vi "Set Error.vi"(4 "Log Error?":bool, 6 "Error Message":string, 7 "Error Codes":T1) -> (3 "Error Interface out":refnum<class "Error Interface.lvclass">)   [LabVIEW 2016, in "Stream Error.lvlib" / "Error Interface.lvclass"]
doc: "--\nCopyright © 2017 Composed SystemsI All rights reserved.\n\nAuthor: Jon McBee <jon.mcbee@composed.io>\n\nThis library is provided \"AS IS\" ,WITHOUT WARRANTIES OR\nCONDITIONS OF ANY KIND, either express or implied.\n\nComposed Systems -- composed.io\n\nStream 0.0.1.1\nJon McBee - Composed Systems\nCopyright (c) 2017, Composed Systems"
uses:
  <userlib>/Composed Systems/Stream/Error/Classes/Error Interface/Error Interface.lvclass
  <userlib>/Composed Systems/Stream/Error/Classes/Error Interface/Error Codes.ctl
  <userlib>/Composed Systems/Stream/Error/Classes/Error Interface/Error Interface.lvclass/Error Interface.ctl
  <userlib>/Composed Systems/Stream/Log/Application Log/Log Level.ctl
  <userlib>/Composed Systems/Stream/Log/Global Application Log/Global Application Log.lvclass
  <userlib>/Composed Systems/Stream/Log/Application Log/Application Log.lvclass
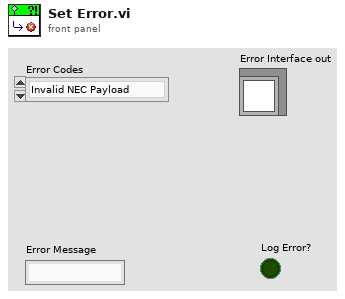
[diagram p1: front panel]
types:
  T1 = typedef "Stream Error.lvlib/Error Interface.lvclass/Error Codes.ctl" = enum16{"Invalid NEC Payload"}
  T2 = typedef "Stream Log.lvlib/Application Log.lvclass/Log Level.ctl" = enum16{"Imperative", "Major", "Minor", "Debug", "Off"}
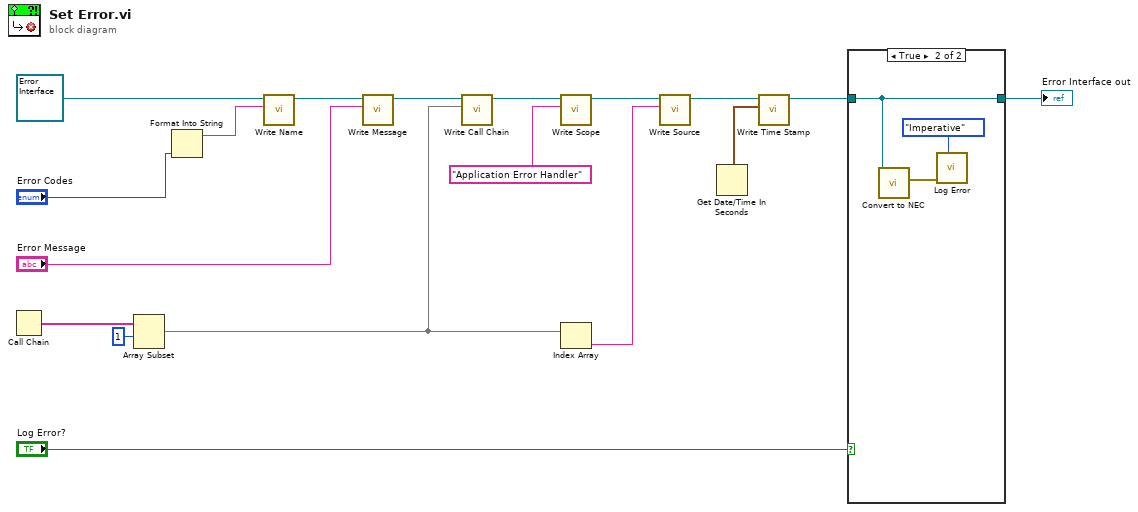
[diagram p0: block diagram]
diagram:
  n1 = Call Chain() -> (call chain=w9:string[])
  n2 = Array Subset(array=w9, index=1) -> (w5:string[])  [unwired: 1 in]
  n3 = Format Into String("Error Codes") -> (resulting string=w15:string)  [unwired: 3 in, 1 out]
  n4 = call <userlib>:"Write Name.vi"("Name"=w15, "Error Interface in"=refnum<class "Error Interface.lvclass"> refnum ("Error Interface out")) -> ("Error Interface out"=w17:refnum<class "Error Interface.lvclass">)  [unwired: 8 in, 1 out]
  n5 = call <userlib>:"Write Message.vi"("Message"="Error Message", "Error Interface in"=w17) -> ("Error Interface out"=w13:refnum<class "Error Interface.lvclass">)  [unwired: 8 in, 1 out]
  n6 = call <userlib>:"Write Call Chain.vi"("Call Chain"=w5, "Error Interface in"=w13) -> ("Error Interface out"=w12:refnum<class "Error Interface.lvclass">)  [unwired: 8 in, 1 out]
  n7 = call <userlib>:"Write Scope.vi"("Scope"="Application Error Handler", "Error Interface in"=w12) -> ("Error Interface out"=w11:refnum<class "Error Interface.lvclass">)  [unwired: 8 in, 1 out]
  n8 = Index Array(array=w5) -> (element=w4:string)  [unwired: 1 in]
  n9 = call <userlib>:"Write Source.vi"("Source"=w4, "Error Interface in"=w11) -> ("Error Interface out"=w10:refnum<class "Error Interface.lvclass">)  [unwired: 8 in, 1 out]
  n10 = Get Date/Time In Seconds() -> (seconds since 1Jan1904=w7:timestamp)
  n11 = call <userlib>:"Write Time Stamp.vi"("Time Stamp"=w7, "Error Interface in"=w10) -> ("Error Interface out"=w2:refnum<class "Error Interface.lvclass">)  [unwired: 8 in, 1 out]
  n12 = case shown="True" "Log Error?" {
    tunnel: [w19 w22] -> w1
    tunnel: w2 -> [w19 w22]
    frame False {
    }
    frame True {
      n13 = call <userlib>:"Convert to NEC.vi"("Error Interface in"=w22) -> ("error out"=w21:errorcluster)  [unwired: 10 in]
      n14 = call <userlib>:"Log Error.vi"("Level"=Log_Level."Imperative", "error in (no error)"=w21) -> ()  [unwired: 9 in, 1 out]
    }
  }
  "Error Interface out" <- w1
